vi "hourly - Copy.vi"(8 "error in (no error)":errorcluster) -> (0 "error out":errorcluster)   [LabVIEW 2017]
uses:
  <vilib>/Math Plots/3D Math Plots/3D Pie/3D Pie XCtrl/3D Pie.xctl
  <vilib>/addons/database/Connection.llb/DB Tools Open Connec (Path).vi
  <vilib>/addons/database/Connection.llb/Conn Execute.vi
  <vilib>/addons/database/Recordset.llb/Rec Fetch Recordset Data (R).vi
  <vilib>/addons/database/Recordset.llb/Rec Destroy - Connection.vi
  <vilib>/Math Plots/3D Math Plots/3D Pie/3D Pie Datatype/Public/Plot Helper (Vector).vi
  <vilib>/addons/database/NI_Database_API.lvlib
  <vilib>/Math Plots/3D Math Plots/3D Pie/3D Pie Datatype/3D Pie Datatype.lvclass
panel:
  out "Station list":string[](array[string])
  out "Station size":i32
  in  "Tab Control":T1(tab)
  out "Table":string[][](table)
  out "Production":refnum<class "3D Plot Datatype.lvclass">[](xcontrol)
  out "Rejection":refnum<class "3D Plot Datatype.lvclass">[](xcontrol)
  out "Station Count":i32
  out "All Shifts":bool
  in  "Cancel Button - Archive":bool
  in  "Download 2":bool
  in  "Get Rport 2":bool
  in  "Shift":string(combo)
  in  "Station":string(combo)
  in  "Date":timestamp format="%<%Y-%m-%d>T"
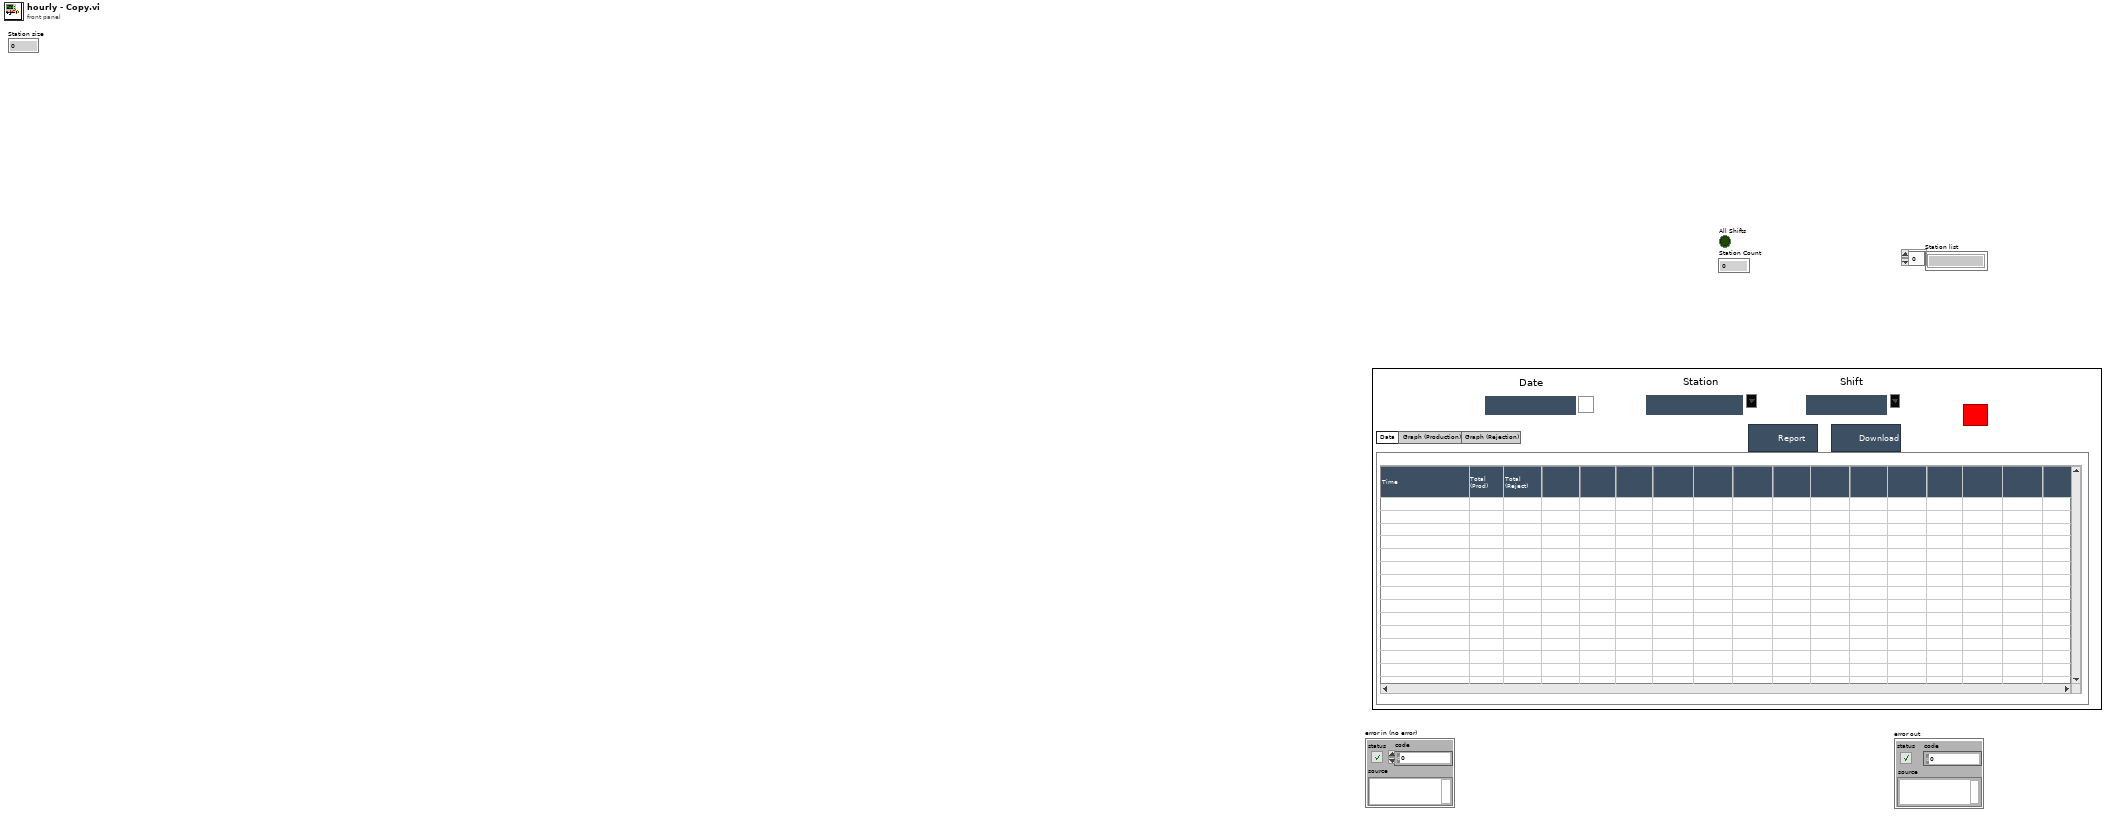
[diagram p1: front panel]
types:
  T1 = enum32{"Data", "Graph (Production)", "Graph (Rejection)"}
  T2 = typedef "NI_Database_API.lvlib/Conn ObjectReference.ctl" = refnum<k1>
  T3 = typedef "NI_Database_API.lvlib/Rec ObjectReference.ctl" = refnum<k1>
  T4 = enum32{"invalid app kind", "Development System", "Run Time System", "Student Edition", "Embedded LabVIEW", "Evaluation", "Custom"}
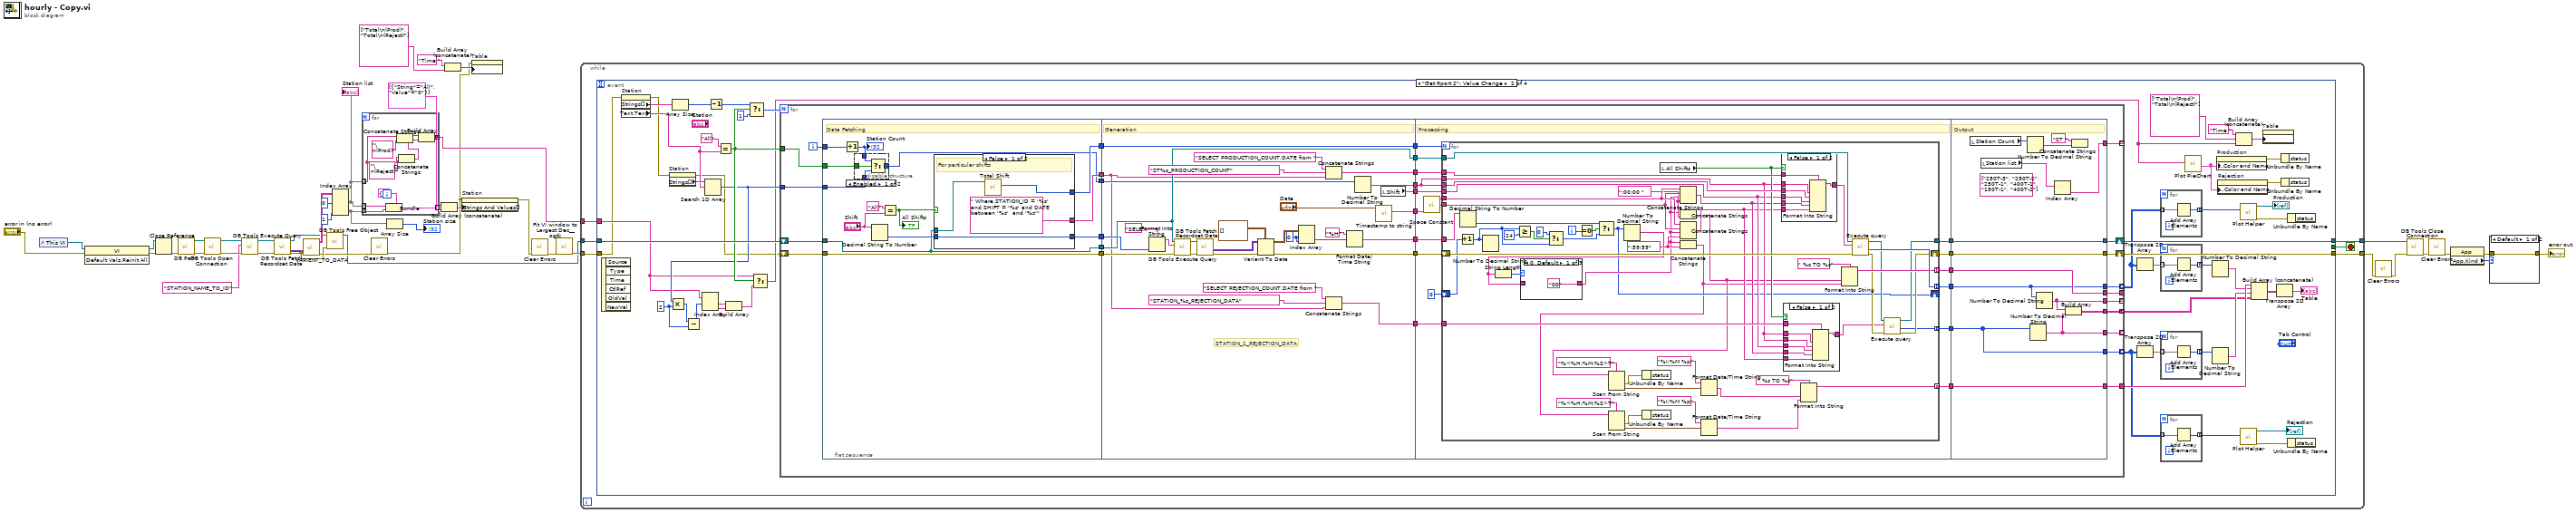
[diagram p0: block diagram]
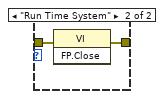
[diagram p2: hidden frame]
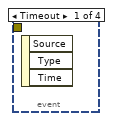
[diagram p3: hidden frame]
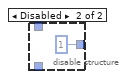
[diagram p4: hidden frame]
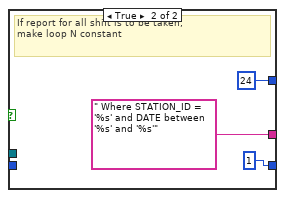
[diagram p5: hidden frame]
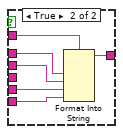
[diagram p6: hidden frame]
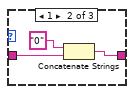
[diagram p7: hidden frame]
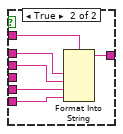
[diagram p9: hidden frame]
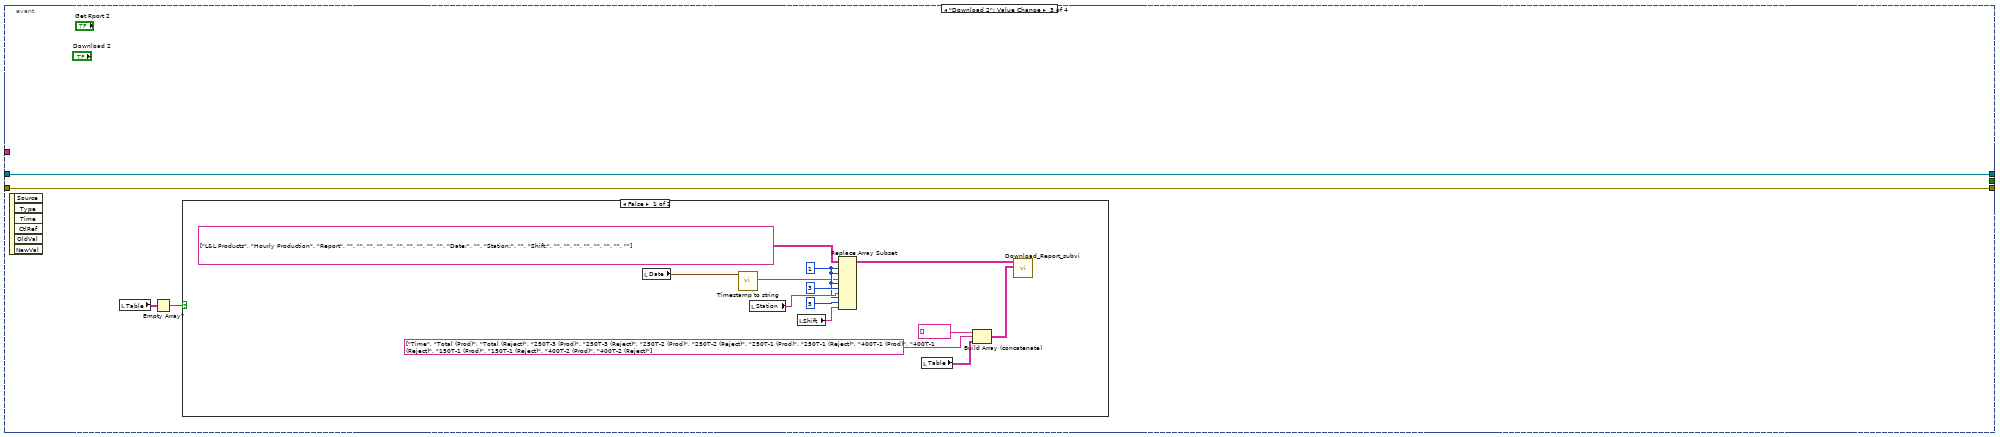
[diagram p10: hidden frame]
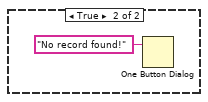
[diagram p11: hidden frame]
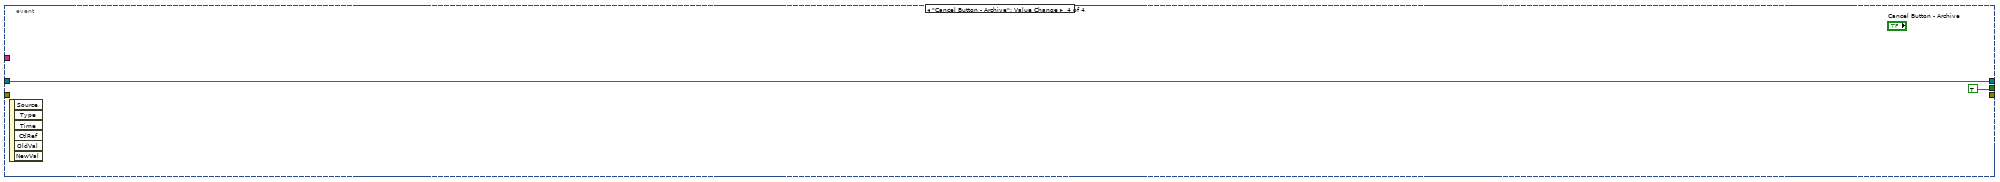
[diagram p12: hidden frame]
diagram:
  n1 = control-ref of="This VI"() -> (w36:refnum<vi>)
  n2 = invoke class="VI" method="Default Vals.Reinit All"(reference=w36, error in="error in (no error)") -> (reference out=w34:refnum<vi>, error out=w35:errorcluster)  [unwired: 1 in, 1 out]
  n3 = Close Reference(reference=w34, error in (no error)=w35) -> (error out=w33:errorcluster)
  n4 = call "DB Path.vi"("error in"=w33) -> ("error out"=w32:errorcluster, "DB Path"=w31:path)  [unwired: 9 in]
  n5 = call-poly <vilib>:"DB Tools Open Connection.vi"("error in (no error)"=w32, "connection information"=w31) -> ("error out"=w20:errorcluster, "connection reference"=w21:T2)  [unwired: 6 in]
  n6 = call-poly <vilib>:"DB Tools Execute Query.vi"("error in (no error)"=w20, "SQL query"="STATION_NAME_TO_ID", "connection reference"=w21) -> ("error out"=w29:errorcluster, "recordset reference"=w30:T3)  [unwired: 5 in]
  n7 = call-poly <vilib>:"DB Tools Fetch Recordset Data.vi"("error in (no error)"=w29, "recordset reference"=w30) -> ("error out"=w24:errorcluster, "recordset data"=w28:variant[][], "recordset reference out"=w22:T3)  [unwired: 3 in]
  n8 = call "VARIENT_TO_DATA.vi"("data"=w28, "error in (no error)"=w24) -> ("Table"=w25:string[][], "error out"=w23:errorcluster)  [unwired: 7 in]
  n9 = call-poly <vilib>:"DB Tools Free Object.vi"("error in (no error)"=w24, "recordset reference"=w22) -> ("connection reference"=w9:T2)  [unwired: 8 in, 1 out]
  n10 = Index Array(array=w25, index (col) #1=0 ("index (row)"), index (col) #2=1 ("index (col)")) -> (element #1=w8:string[], element #2=w15:string[])  [unwired: 2 in]
  "Station list" <- w8
  n11 = for {
    tunnel: w8 -> [w52] mode=indexing
    tunnel: w15 -> [w51] mode=indexing
    tunnel: [w49] -> w16 mode=indexing
    tunnel: w8 -> [w46] mode=indexing
    tunnel: [w43] -> w7 mode=concatenating
    n12 = Bundle(cluster=cluster{"String":string, "Value":string} {"String"="", "Value"=""}, "String"=w52, "Value"=w51) -> (w49:cluster{"String":string, "Value":string})
    n13 = Concatenate Strings(w46, "\n(Prod)" ("string")) -> (w44:string)
    n14 = Concatenate Strings(w46, "\n(Reject)" ("string")) -> (w45:string)
    n15 = Build Array(w44, w45) -> (w43:string[])
  }
  n16 = call <vilib>:"Clear Errors.vi"("error in (no error)"=w23) -> ("error out"=w1:errorcluster)  [unwired: 5 in, 1 out]
  n17 = Array Size(array=w15) -> (size(s)=→"Station size":i32)
  n18 = Build Array (concatenate)(cluster{"String":string, "Value":string}[] [{"String"="All", "Value"="0"}] ("array"), w16) -> (w18:cluster{"String":string, "Value":string}[])
  n19 = Build Array (concatenate)("Time ", string[] ["Total\n(Prod)", "Total\n(Reject)"]) -> (w2:string[])
  n20 = property on="Station" class="CmbBox"(error in=w1, "Strings And Values[]"=w18) -> (error out=w12:errorcluster)  [unwired: 1 in, 1 out]
  n21 = property on="Table" class="Tbl (strict)"(error in=w1, "Column Headers[]"=w2) -> ()  [unwired: 1 in, 2 out]
  n22 = call <vilib>:"Clear Errors.vi"("error in (no error)"=w12) -> ("error out"=w13:errorcluster)  [unwired: 5 in, 1 out]
  n23 = call <userlib>:"Fit VI window to Largest Dec__ogtk.vi"("error in (no error)"=w13) -> ("error out"=w10:errorcluster)  [unwired: 5 in, 1 out]
  n24 = while {
    tunnel: w10 -> [w55]
    tunnel: w9 -> [w54]
    tunnel: [w57] -> w5
    tunnel: [w56] -> w38
    tunnel: w7 -> [w53]
    stop <- w58 stop-if-true
    n25 = event shown="[1] \"Get Rport 2\": Value Change" {
      selector: _ -> [_ _ _ _]
      dyn-events: _ -> [_ _ _ _]
      timeout: _ -> [_ _ _ _]
      tunnel: w54 -> [_ w106 w323 w338]
      tunnel: [_ _ _ TRUE] -> w58
      tunnel: [_ w104 w322 _] -> w57
      tunnel: [_ w105 w323 w338] -> w56
      tunnel: w55 -> [_ w60 w322 _]
      tunnel: w53 -> [_ w85 _ _]
      event Timeout {
        n26 = event-data() -> ()  [unwired: 1 in, 3 out]
      }
      event "Get Rport 2": Value Change {
        w88 = 2 ("y")
        n27 = event-data() -> ()  [unwired: 1 in, 6 out]
        n28 = property on="Station" class="CmbBox"(error in=w60) -> (error out=w61:errorcluster, "Strings[]"=w100:string[], "Text.Text"=w62:string)  [unwired: 1 in, 1 out]
        n29 = property on="Station" class="CmbBox"(error in=w61) -> (error out=w59:errorcluster, "Strings[]"=w97:string[])  [unwired: 1 in, 1 out]
        n30 = Array Size(array=w100) -> (size(s)=w99:i32)
        n31 = Search 1D Array(1D array=w97, element=w62) -> (index of element=w92:i32)  [unwired: 1 in]
        n32 = Multiply(x=w92, y=w88) -> (x*y=w87:i32)
        n33 = Subtract(x=w87, y=w88) -> (x-y=w86:i32)
        n34 = Index Array(array=w85, index #1=w86) -> (element #1=w90:string, element #2=w91:string)  [unwired: 1 in]
        n35 = Decrement(x=w99) -> (x-1=w98:i32)
        n36 = Equal?(x="All", y=w62) -> (x = y?=w93:bool)
        n37 = Build Array(w90, w91) -> (w89:string[])
        n38 = Select(t=w98, s=w93, f=1) -> (s? t:f=w102:i32)
        n39 = Select(t=w85, s=w93, f=w89) -> (s? t:f=w83:string[])
        n40 = for {
          N: w102 -> [_]
          shift-right: [w131] -> w105
          shift-left: w106 -> [w132]
          shift-right: [w130] -> w104
          shift-left: w59 -> [w129]
          tunnel: w93 -> [w128]
          tunnel: w92 -> [w127]
          tunnel: [w124] -> _
          tunnel: [w125] -> _ mode=indexing
          tunnel: [w123] -> _ mode=indexing
          tunnel: [w122] -> w66 mode=indexing
          tunnel: [w119] -> _ mode=indexing
          tunnel: [w118] -> w70 mode=concatenating
          tunnel: [w117] -> w78
          tunnel: [w115] -> w65 mode=indexing
          i -> [w126]
          n41 = flat-sequence {
            tunnel: w129 -> [w164]
            tunnel: w132 -> [w156]
            tunnel: [w162] -> w150
            tunnel: [w163] -> w149
            tunnel: [w164] -> w148
            tunnel: [w156] -> w147
            tunnel: [w151] -> w146
            tunnel: [w158] -> w145
            tunnel: w128 -> [w155]
            tunnel: w127 -> [w154]
            tunnel: w126 -> [w153]
            tunnel: [w199] -> w144
            tunnel: [w181] -> w143
            tunnel: [w197] -> w142
            tunnel: [w205] -> w141
            tunnel: [w204] -> w140
            tunnel: [w203] -> w139
            tunnel: [w195] -> w138
            tunnel: [w202] -> w137
            tunnel: w145 -> [w183]
            tunnel: w146 -> [w184]
            tunnel: w147 -> [w203]
            tunnel: w148 -> [w187]
            tunnel: w149 -> [w178]
            tunnel: w150 -> [w202]
            tunnel: [w177] -> w121
            tunnel: [w220] -> w136
            tunnel: [w217] -> w135
            tunnel: [w214] -> w134
            tunnel: [w213] -> w133
            tunnel: w144 -> [w221]
            tunnel: w143 -> [w218]
            tunnel: w142 -> [w216]
            tunnel: w141 -> [w215]
            tunnel: w140 -> [w210]
            tunnel: w139 -> [w212]
            tunnel: w138 -> [w211]
            tunnel: w137 -> [w207]
            tunnel: w121 -> [w209]
            tunnel: [w208] -> w120
            tunnel: [w206] -> w116
            tunnel: [w319] -> w131
            tunnel: w136 -> [w318]
            tunnel: w135 -> [w319]
            tunnel: w134 -> [w308]
            tunnel: w133 -> [w313]
            tunnel: [w318] -> w130
            tunnel: [w312] -> w125
            tunnel: [w313] -> w124
            tunnel: [w314] -> w123
            tunnel: [w308] -> w122
            tunnel: w120 -> [w307]
            tunnel: [w311] -> w119
            tunnel: [w310] -> w118
            tunnel: [w309] -> w117
            tunnel: w116 -> [w309]
            tunnel: [w307] -> w115
            frame #0 {
              # "Data Fetching"
              n42 = Increment(x=w153) -> (x+1=w152:i32)
              "Station Count" <- w152
              n43 = disable-structure shown="Enabled" {
                disable-tunnel: w155 -> [w168 _]
                disable-tunnel: w154 -> [w167 _]
                disable-tunnel: w152 -> [w166 _]
                disable-tunnel: [w165 1 ("index of element")] -> w151
                frame Enabled {
                  n44 = Select(t=w166, s=w168, f=w167) -> (s? t:f=w165:i32)
                }
                frame Disabled {
                }
              }
              n45 = Decimal String To Number(string="Shift") -> (number=w157:i32)  [unwired: 2 in, 1 out]
              n46 = Equal?(x="All", y="Shift") -> (x = y?=w160:bool)
              "All Shifts" <- w160
              n47 = case shown="False" w160 {
                tunnel: [" Where STATION_ID = '%s' and SHIFT = '%s' and DATE between '%s'  and '%s'" ("format string") " Where STATION_ID = '%s' and DATE between '%s' and '%s'" ("format string")] -> w163
                tunnel: w156 -> [w172 _]
                tunnel: [w171 24 ("Shift Hrs")] -> w162
                tunnel: [w170 1] -> w158
                tunnel: w157 -> [w170 _]
                frame False {
                  # "For particular shifts"
                  n48 = call "Total Shift.vi"("connection reference"=w172) -> ("Shift Hrs"=w171:i32)  [unwired: 9 in, 1 out]
                }
                frame True {
                  # "If report for all shift is to be taken,\nmake loop N constant"
                }
              }
            }
            frame #1 {
              w191 = 0 ("index (row)")
              # "STATION_1_REJECTION_DATA"
              # "Generation"
              n49 = Format Into String(format string="SELECT SHIFT_START FROM master_shift WHERE SHIFT_ID = %d  " ("SQL query"), w183) -> (resulting string=w189:string)  [unwired: 2 in, 1 out]
              n50 = call-poly <vilib>:"DB Tools Execute Query.vi"("error in (no error)"=w187, "SQL query"=w189, "connection reference"=w203) -> ("error out"=w186:errorcluster, "recordset reference"=w185:T3)  [unwired: 5 in]
              n51 = call-poly <vilib>:"DB Tools Fetch Recordset Data.vi"("error in (no error)"=w186, "recordset reference"=w185) -> ("error out"=w194:errorcluster, "recordset data"=w192:variant[][])  [unwired: 3 in, 1 out]
              n52 = Variant To Data(error in=w194, type=timestamp[][] [] ("From Date 2"), Variant=w192) -> (data=w193:timestamp[][], error out=w205:errorcluster)
              n53 = Index Array(array=w193, index (row)=w191, index (col)=w191) -> (element=w198:timestamp)
              n54 = Concatenate Strings("SELECT PRODUCTION_COUNT,DATE from " ("format string"), "ST%s_PRODUCTION_COUNT", w178) -> (w199:string)
              n55 = Concatenate Strings("SELECT REJECTION_COUNT,DATE from " ("format string"), "STATION_%s_REJECTION_DATA", w178) -> (w177:string)
              n56 = Format Date/Time String(time format string (%c)="%H", seconds (now)=w198) -> (date/time string=w197:string)  [unwired: 1 in]
              n57 = Number To Decimal String(number=w184) -> (decimal integer string=w204:string)  [unwired: 1 in]
              n58 = call "Timestamp to string.vi"("time stamp"="Date") -> ("Date"=w181:string)  [unwired: 8 in, 2 out]
              n59 = local read "Shift"() -> (w195:string)
            }
            frame #2 {
              # "Processing"
              n60 = call <vilib>:"Space Constant.vi"() -> ("String"=w222:string)
              n61 = for {
                N: w207 -> [_]
                tunnel: w221 -> [w274]
                tunnel: w218 -> [w264]
                tunnel: w222 -> [w259]
                tunnel: w212 -> [w257]
                tunnel: w211 -> [w243]
                tunnel: w210 -> [w255]
                shift-right: [w239] -> _
                shift-left: 0 -> [w269]
                tunnel: w216 -> [w263]
                tunnel: [w262] -> w214 mode=indexing
                tunnel: [w260] -> w213 mode=indexing
                tunnel: [w247] -> w217
                shift-right: [w248] -> w220
                shift-left: w215 -> [w273]
                tunnel: w210 -> [w244]
                tunnel: w209 -> [w245]
                tunnel: [w240] -> w208 mode=indexing
                tunnel: [w224] -> w206 mode=indexing
                i -> [w272]
                w256 = ":00:00 " ("input 2")
                w258 = ":59:59" ("input 2")
                n62 = Decimal String To Number(string=w263) -> (number=w270:i32)  [unwired: 2 in, 1 out]
                n63 = Increment(x=w269) -> (x+1=w254:i32)
                n64 = Number To Decimal String(number=w254) -> ()  [unwired: 1 in, 1 out]
                n65 = Greater Or Equal?(x=w254, y=24) -> (x >= y?=w267:bool)
                n66 = Select(t=0 ("y"), s=w267, f=w254) -> (s? t:f=w265:i32)
                n67 = Equal To 0?(x=w272) -> (x = 0?=w271:bool)
                n68 = Select(t=w270, s=w271, f=w265) -> (s? t:f=w239:i32)
                n69 = Number To Decimal String(number=w239) -> (decimal integer string=w251:string)  [unwired: 1 in]
                n70 = String Length(string=w251) -> (length=w253:i32)
                n71 = case shown="0, Default" w253 {
                  tunnel: ["00" w290 w292] -> w252
                  tunnel: w251 -> [_ w289 w292]
                  frame 0, Default {
                  }
                  frame 1 {
                    n72 = Concatenate Strings("0", w289) -> (w290:string)
                  }
                  frame 2 {
                  }
                }
                n73 = local read "All Shifts"() -> (w246:bool)
                n74 = Concatenate Strings(w264, w259, w252, w256) -> (w242:string)
                n75 = Concatenate Strings(w252, w256) -> (w233:string)
                n76 = Scan From String(format string="%<%H:%M:%S>T", input string=w233) -> (error out=w232:errorcluster, output 1=w234:timestamp)  [unwired: 3 in, 2 out]
                n77 = Unbundle By Name(w232) -> ()  [unwired: 1 out]
                n78 = Concatenate Strings(w264, w259, w252, w258) -> (w241:string)
                n79 = Concatenate Strings(w252, w258) -> (w223:string)
                n80 = Scan From String(format string="%<%H:%M:%S>T", input string=w223) -> (error out=w228:errorcluster, output 1=w227:timestamp)  [unwired: 3 in, 2 out]
                n81 = Unbundle By Name(w228) -> ()  [unwired: 1 out]
                n82 = Format Date/Time String(time format string (%c)="%I:%M %p" ("format string"), seconds (now)=w234) -> (date/time string=w230:string)  [unwired: 1 in]
                n83 = Format Date/Time String(time format string (%c)="%I:%M %p" ("format string"), seconds (now)=w227) -> (date/time string=w225:string)  [unwired: 1 in]
                n84 = case shown="False" w246 {
                  tunnel: w274 -> [w299 w305]
                  tunnel: [w298 w304] -> w238
                  tunnel: w243 -> [w297 _]
                  tunnel: w242 -> [w296 w303]
                  tunnel: w241 -> [w295 w302]
                  tunnel: w255 -> [w294 w301]
                  tunnel: w244 -> [w293 w300]
                  frame False {
                    n85 = Format Into String(format string=w299, w293, w294, w297, w296, w295) -> (resulting string=w298:string)  [unwired: 2 in, 1 out]
                  }
                  frame True {
                    n86 = Format Into String(format string=w305, w300, w301, w303, w302) -> (resulting string=w304:string)  [unwired: 2 in, 1 out]
                  }
                }
                n87 = case shown="False" w246 {
                  tunnel: w245 -> [w281 w287]
                  tunnel: [w280 w286] -> w237
                  tunnel: w243 -> [w279 _]
                  tunnel: w242 -> [w278 w285]
                  tunnel: w241 -> [w277 w284]
                  tunnel: w244 -> [w276 w283]
                  tunnel: w244 -> [w275 w282]
                  frame False {
                    n88 = Format Into String(format string=w281, w275, w276, w279, w278, w277) -> (resulting string=w280:string)  [unwired: 2 in, 1 out]
                  }
                  frame True {
                    n89 = Format Into String(format string=w287, w282, w283, w285, w284) -> (resulting string=w286:string)  [unwired: 2 in, 1 out]
                  }
                }
                n90 = Format Into String(format string=" %s TO %s", w230, w225) -> (resulting string=w224:string)  [unwired: 2 in, 1 out]
                n91 = Format Into String(format string=" %s TO %s", w233, w223) -> (resulting string=w260:string)  [unwired: 2 in, 1 out]
                n92 = call "Execute query.vi"("error in (no error)"=w273, "String"=w238, "connection reference"=w257) -> ("error out"=w249:errorcluster, "Production Count"=w262:i32, "connection reference 2"=w250:T2)  [unwired: 3 in, 3 out]
                n93 = call "Execute query.vi"("error in (no error)"=w249, "String"=w237, "connection reference"=w250) -> ("error out"=w248:errorcluster, "Production Count"=w240:i32, "connection reference 2"=w247:T2)  [unwired: 3 in, 3 out]
              }
            }
            frame #3 {
              (unwired) string[] ["250T-3", "250T-2", "250T-1", "400T-1", "150T-1", "400T-2"]
              # "Output"
              n94 = local read "Station Count"() -> (w315:i32)
              n95 = local read "Station list"() -> (w306:string[])
              n96 = Number To Decimal String(number=w315) -> (decimal integer string=w316:string)  [unwired: 1 in]
              n97 = Number To Decimal String(number=w307) -> (decimal integer string=w311:string[])  [unwired: 1 in]
              n98 = Number To Decimal String(number=w308) -> (decimal integer string=w312:string[])  [unwired: 1 in]
              n99 = Index Array(array=w306) -> (element=w314:string)  [unwired: 1 in]
              n100 = Build Array(w312, w311) -> (w310:string[][])
              n101 = Concatenate Strings("ST " ("string"), w316) -> ()  [unwired: 1 out]
            }
          }
        }
        n102 = Transpose 2D Array(2D array=w66) -> (transposed array=w74:i32[][])
        n103 = Transpose 2D Array(2D array=w65) -> (transposed array=w73:i32[][])
        n104 = for {
          tunnel: w66 -> [w114] mode=indexing
          tunnel: [w113] -> w77 mode=indexing
          n105 = Add Array Elements(numeric array=w114) -> (sum=w113:i32)
        }
        n106 = for {
          tunnel: w74 -> [w112] mode=indexing
          tunnel: [w111] -> w75 mode=indexing
          n107 = Add Array Elements(numeric array=w112) -> (sum=w111:i32)
        }
        n108 = for {
          tunnel: w73 -> [w110] mode=indexing
          tunnel: [w109] -> w72 mode=indexing
          n109 = Add Array Elements(numeric array=w110) -> (sum=w109:i32)
        }
        n110 = for {
          tunnel: w65 -> [w108] mode=indexing
          tunnel: [w107] -> w69 mode=indexing
          n111 = Add Array Elements(numeric array=w108) -> (sum=w107:i32)
        }
        n112 = call "Plot PieChart.vi"("Label"=w83) -> ("Labelling"=w63:cluster{dbl, "String":string}[])  [unwired: 10 in]
        n113 = Number To Decimal String(number=w75) -> (decimal integer string=w76:string[])  [unwired: 1 in]
        n114 = Number To Decimal String(number=w72) -> (decimal integer string=w71:string[])  [unwired: 1 in]
        n115 = property on="Production" class="3D Pie (strict)"("Plot Specific:Color and Name"=w63) -> (error out=w81:errorcluster)  [unwired: 2 in, 1 out]
        n116 = property on="Rejection" class="3D Pie (strict)"("Plot Specific:Color and Name"=w63) -> (error out=w64:errorcluster)  [unwired: 2 in, 1 out]
        n117 = Build Array (concatenate)("Time ", string[] ["Total\n(Prod)", "Total\n(Reject)"], w83) -> (w94:string[])
        n118 = call-poly <vilib>:"Plot Helper.vi"("x vector"=w77) -> ("error out"=w84:errorcluster, "3D Plot lvclass Array out"=→"Production":refnum<class "3D Plot Datatype.lvclass">[])  [unwired: 2 in, 7 out]
        n119 = call-poly <vilib>:"Plot Helper.vi"("x vector"=w69) -> ("error out"=w68:errorcluster, "3D Plot lvclass Array out"=→"Rejection":refnum<class "3D Plot Datatype.lvclass">[])  [unwired: 2 in, 7 out]
        n120 = Build Array (concatenate)(w78, w76, w71, w70) -> (w95:string[][])
        n121 = property on="Table" class="Tbl (strict)"("Column Headers[]"=w94) -> ()  [unwired: 2 in, 2 out]
        n122 = Transpose 2D Array(2D array=w95) -> (transposed array=→"Table":string[][])
        n123 = Unbundle By Name(w81) -> ()  [unwired: 1 out]
        n124 = Unbundle By Name(w64) -> ()  [unwired: 1 out]
        n125 = Unbundle By Name(w84) -> ()  [unwired: 1 out]
        n126 = Unbundle By Name(w68) -> ()  [unwired: 1 out]
      }
      event "Download 2": Value Change {
        n127 = event-data() -> ()  [unwired: 1 in, 6 out]
        n128 = local read "Table"() -> (w321:string[][])
        n129 = Empty Array?(array=w321) -> (empty?=w320:bool)
        n130 = case shown="False" w320 {
          frame False {
            w332 = 1 ("index (row)")
            n131 = local read "Date"() -> (w329:timestamp)
            n132 = call "Timestamp to string.vi"("time stamp"=w329) -> ("Date"=w328:string)  [unwired: 8 in, 2 out]
            n133 = local read "Station"() -> (w333:string)
            n134 = local read "Shift"() -> (w330:string)
            n135 = Replace Array Subset(array=string[][] [["L&L Products", "Hourly Production", "Report", "", "", "", "", "", "", "", "", "", ""], ["Date:", "", "Station:", "", "Shift:", "", "", "", "", "", "", "", ""]] ("Column Header Strings[]"), new element #1=w328, index (row) #1=w332, index (col) #1=w332, new element #2=w333, index (row) #2=w332, index (col) #2=3 ("disabled index (col)"), new element #3=w330, index (row) #3=w332, index (col) #3=5 ("disabled index (col)")) -> (w335:string[][])
            n136 = local read "Table"() -> (w326:string[][])
            n137 = Build Array (concatenate)(string[] [] ("element"), string[] ["Time", "Total (Prod)", "Total (Reject)", "250T-3 (Prod)", "250T-3 (Reject)", "250T-2 (Prod)", "250T-2 (Reject)", "250T-1 (Prod)", "250T-1 (Reject)", "400T-1 (Prod)", "400T-1 (Reject)", "150T-1 (Prod)", "150T-1 (Reject)", "400T-2 (Prod)", "400T-2 (Reject)"], w326) -> (w325:string[][])
            n138 = call "Download_Report_subvi.vi"("Value"=w325, "Column Header Strings[]"=w335) -> ()  [unwired: 9 in, 1 out]
          }
          frame True {
            n139 = One Button Dialog(message="No record found!") -> ()  [unwired: 1 in, 1 out]
          }
        }
      }
      event "Cancel Button - Archive": Value Change {
        n140 = event-data() -> ()  [unwired: 1 in, 6 out]
      }
    }
  }
  n141 = call <vilib>:"Clear Errors.vi"("error in (no error)"=w5) -> ("error out"=w6:errorcluster)  [unwired: 5 in, 1 out]
  n142 = call <vilib>:"DB Tools Close Connection.vi"("error in (no error)"=w6, "connection reference"=w38) -> ("error out"=w40:errorcluster)  [unwired: 5 in]
  n143 = call <vilib>:"Clear Errors.vi"("error in (no error)"=w40) -> ("error out"=w39:errorcluster)  [unwired: 5 in, 1 out]
  n144 = property class="App"(error in=w39) -> (error out=w41:errorcluster, "App.Kind"=w42:T4)  [unwired: 1 in, 1 out]
  n145 = case shown="Default" w42 {
    tunnel: w41 -> [w340 w342]
    tunnel: [w340 w341] -> w37
    frame Default {
    }
    frame "Run Time System" {
      n146 = invoke class="VI" method="FP.Close"(error in=w342) -> (error out=w341:errorcluster)  [unwired: 2 in, 2 out]
    }
  }
  "error out" <- w37
